vi "Get Buffer.vi"(8 "error in":errorcluster, 11 "Block Upload Sub-Block Transfer in":refnum<class "Block Upload Sub-Block Transfer.lvclass">) -> (0 "error out":errorcluster, 2 "Buffer":map{u8, u8[]}(c390), 3 "Block Upload Sub-Block Transfer out":refnum<class "Block Upload Sub-Block Transfer.lvclass">)   [LabVIEW 2020, in "CANopen.lvlib" / "SDO Manager.lvlib" / "Block Upload Sub-Block Transfer.lvclass"]
uses:
  Block Upload Sub-Block Transfer.lvclass
  Block Upload Sub-Block Transfer.lvclass/Block Upload Sub-Block Transfer.ctl
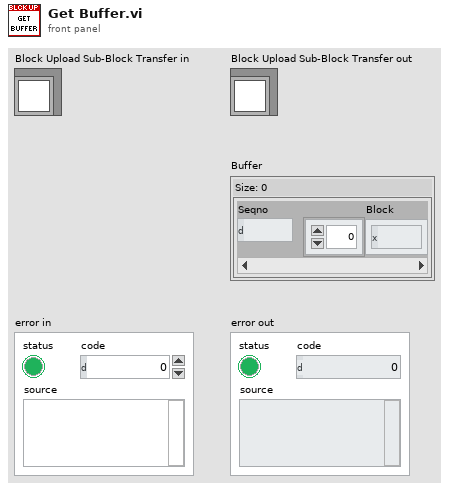
[diagram p1: front panel]
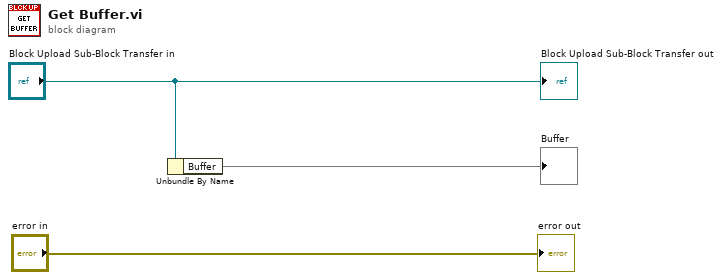
[diagram p0: block diagram]
diagram:
  n1 = Unbundle By Name("Block Upload Sub-Block Transfer in") -> ("Buffer"=→"Buffer":map{u8, u8[]})
  "error out" <- "error in"
  "Block Upload Sub-Block Transfer out" <- "Block Upload Sub-Block Transfer in"
